vi "PBKDF2 Derive Key (Known Salt).vi"(5 "Key length (64 bytes)":i32=64, 7 "HashingAlgorithm (SHA512)":T1=enum."SHA512", 8 "error in (no error)":errorcluster, 9 "iterations (210000)":i32=210000, 10 "Salt":u8[](array[numeric]), 11 "Password":string) -> (0 "error out":errorcluster, 3 "Derived Key":u8[](array[numeric]))   [LabVIEW 2021, in "dotNET Crypto Key Derivation.lvlib"]
doc: "Derive a key from the password using a known salt using the PBKDF2 algorithm.\n\nThis function can be used to validate a previously derived key by using the previously generated salt."
uses:
  dotNET Crypto Key Derivation.lvlib
  Utility/HashingAlgorithm.ctl
  Utility/dotNET Crypto Utility.lvlib
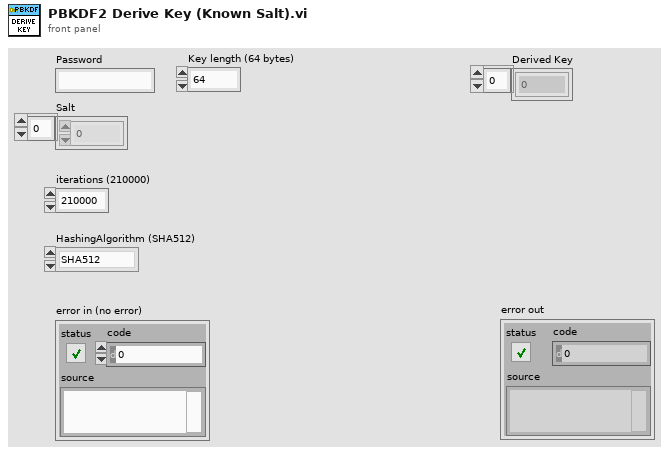
[diagram p1: front panel]
types:
  T1 = typedef "dotNET Crypto Utility.lvlib/HashingAlgorithm.ctl" = enum16{"MD5", "SHA1", "SHA256", "SHA384", "SHA512"}
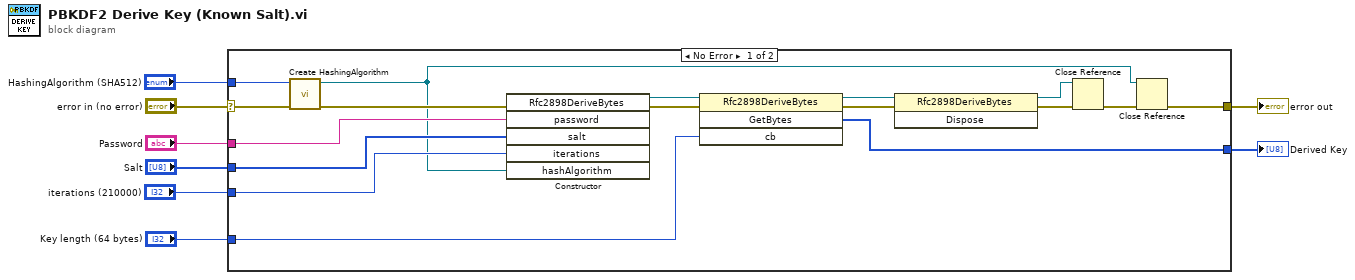
[diagram p0: block diagram]
diagram:
  n1 = case shown="No Error" "error in (no error)" {
    selector: "error in (no error)" -> [w13 w26]
    tunnel: "HashingAlgorithm (SHA512)" -> [w25 _]
    tunnel: "iterations (210000)" -> [w24 _]
    tunnel: "Password" -> [w23 _]
    tunnel: [w22 _] -> w5
    tunnel: "Key length (64 bytes)" -> [w20 _]
    tunnel: [w10 w26] -> w3
    tunnel: "Salt" -> [w12 _]
    frame No Error {
      n2 = call "Create HashingAlgorithm.vi"("error in (no error)"=w13, "HashingAlgorithm"=w25) -> ("error out"=w14:errorcluster, "Hashing Algorithm"=w9:refnum<k24>)  [unwired: 8 in]
      n3 = constructor class="Rfc2898DeriveBytes"(error in=w14, "password"=w23, "salt"=w12, "iterations"=w24, "hashAlgorithm"=w9) -> (reference out=w21:refnum<k24>, error out=w19:errorcluster)  [unwired: 2 in, 5 out]
      n4 = invoke class="Rfc2898DeriveBytes" method="GetBytes"(reference=w21, error in=w19, "cb"=w20) -> (reference out=w17:refnum<k24>, error out=w18:errorcluster, "GetBytes"=w22:u8[])  [unwired: 1 in, 1 out]
      n5 = invoke class="Rfc2898DeriveBytes" method="Dispose"(reference=w17, error in=w18) -> (reference out=w15:refnum<k24>, error out=w16:errorcluster)  [unwired: 1 in, 1 out]
      n6 = Close Reference(reference=w15, error in (no error)=w16) -> (error out=w11:errorcluster)
      n7 = Close Reference(reference=w9, error in (no error)=w11) -> (error out=w10:errorcluster)
    }
    frame Error {
    }
  }
  "Derived Key" <- w5
  "error out" <- w3
